vi "ODMR.vi"() -> ()   [LabVIEW 2017]
uses:
  Expose/Labview/Parameters/ExposeParameterBindingType.ctl
  041ffc80-b207-4d08-bfc5-6ab2d64e676f.vi
  451f70a8-fd5b-4474-9a91-34906ede201c.vi
  76a4058a-f0a1-42dc-85a2-e75da8ad429b.vi
  Experiment/ExpGet.vi
  Expose/Labview/Core/ExposeInvokeMethod.vi
  <userlib>/_OpenG.lib/lvdata/lvdata.llb/Get Default Data from Variant__ogtk.vi
panel:
  in  "btnAbort":bool
  in  "btnRunOdmr":bool
  in  "GateDisplay":cluster{"amp":dbl[][], "dt":dbl}
  in  "Results":T1
  in  "ReaderProperties":cluster{"BinsPerFreq":u32, "MaxFreq":dbl}={"BinsPerFreq"=1, "MaxFreq"=100000.0} caption="Reader" {"MaxFreq" min=0.0 step=0.1; "BinsPerFreq" min=1 max=10000}
  in  "ScanProperties":T2={"Start"=2800.0, "End"=2900.0, "N"=6, "Dwell"=10.0, "StepSize"=20.0, "Amplitude"=-30.0, "RepCount"=3} caption="Scan" {"RepCount" min=1 max=10000000; "StepSize" min=0.0 step=0.1; "Dwell" min=0.0 step=0.1; "N" step=1; "End" min=0.0 step=0.1; "Start" min=0.0 step=0.1}
  out "LastBinIndex":dbl format="%_7g"
  out "PendingRepetitionCount":dbl format="%_7g"
  out "BinIndexIndicator":dbl(slide) max=201.0 step=1.0 scale=0.0..1.0
  out "PendingRepIndcator":dbl(slide) max=3.0 step=1.0 scale=0.0..1.0
  out "IsWorking":bool=TRUE
  out "ExpID":string="Exp967f258c607eed45caf40f4c3101458dC" caption="Exp. ID (Debug)"
  out "Results":dbl[](graph) caption="ODMR"
  in  "ReadTickTime":dbl
  out "Stream":dbl[](graph) caption="Counts"
  out "Digital Waveform Graph":digitalwaveform(graph)
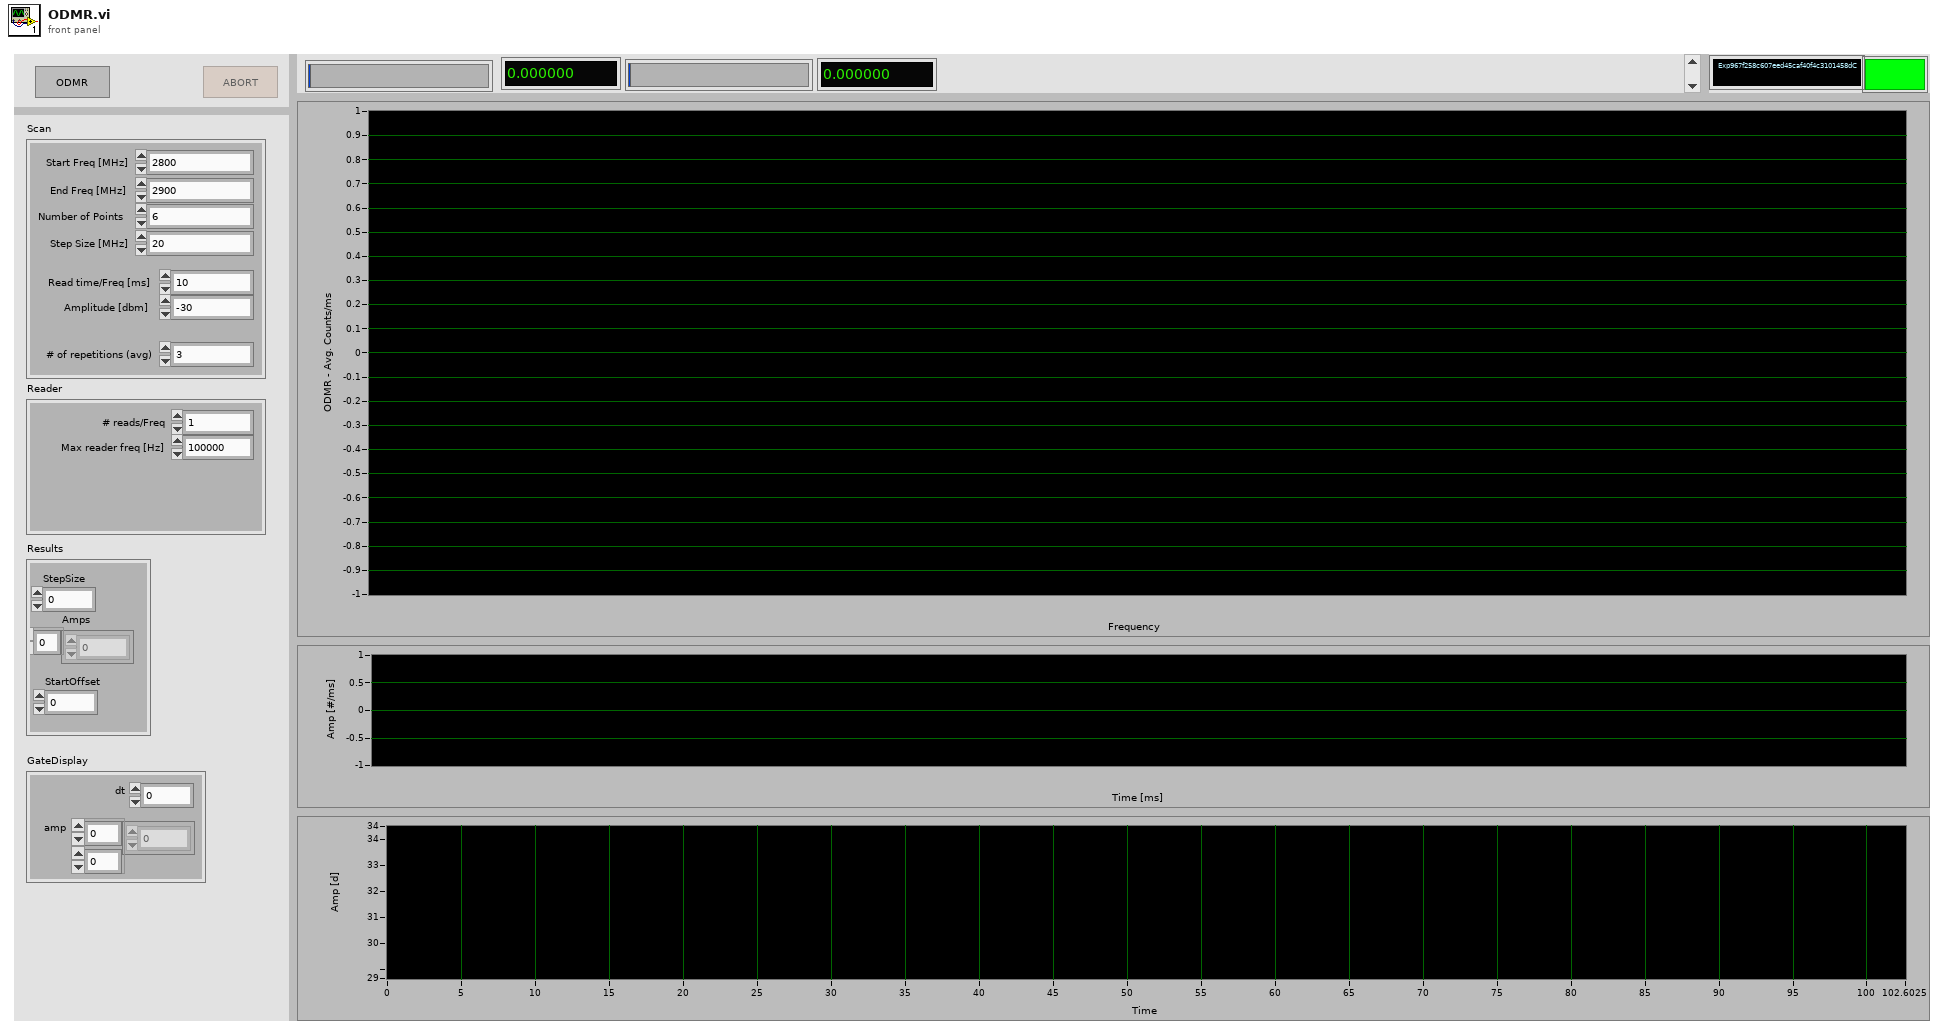
[diagram p1: front panel]
types:
  T1 = cluster{"StepSize":dbl, "Amps":dbl[], "StartOffset":dbl}
  T2 = cluster{"Start":dbl, "End":dbl, "N":u32, "Dwell":dbl, "StepSize":dbl, "Amplitude":dbl, "RepCount":u32}
  T3 = enum8{"Enabled", "Disabled", "Disabled and Grayed Out"}
  T4 = typedef "ExposeParameterBindingType.ctl" = enum16{"ToRemote", "FromRemote", "Bidrectional"}
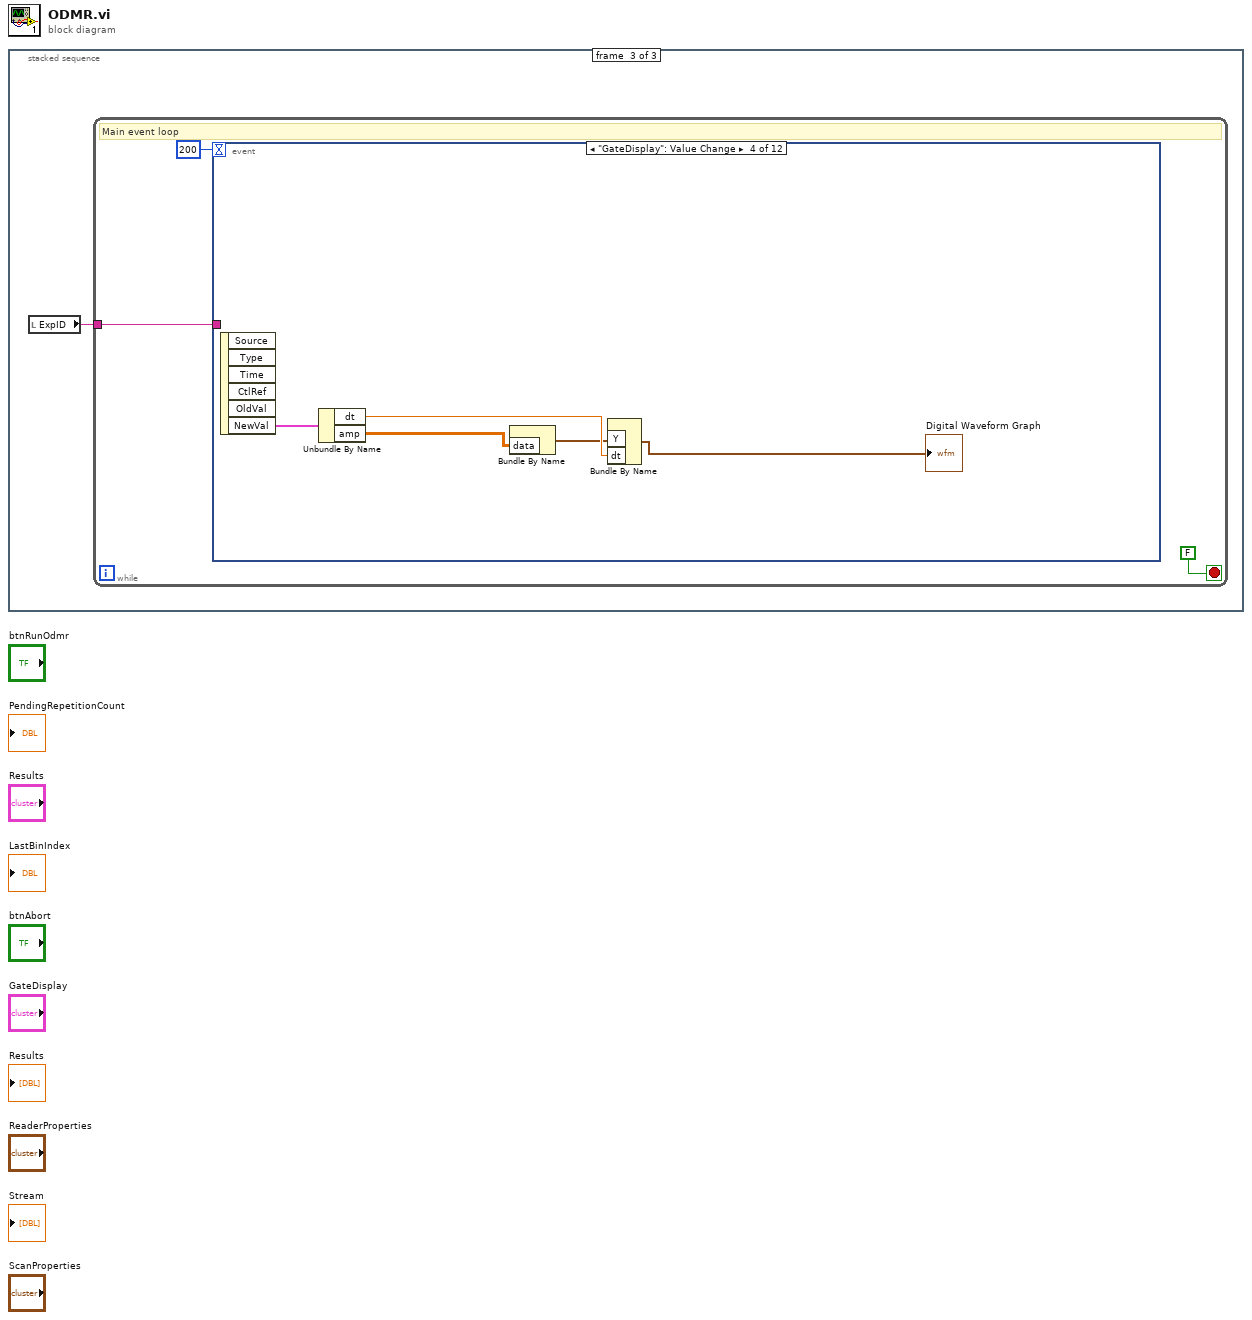
[diagram p0: block diagram]
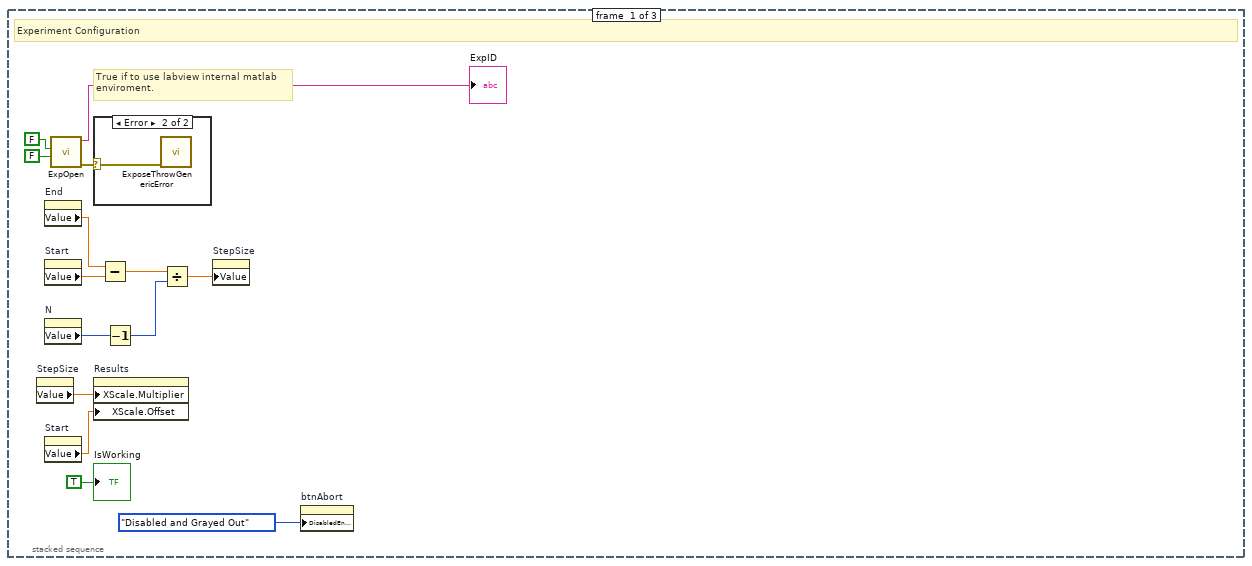
[diagram p2: hidden frame]
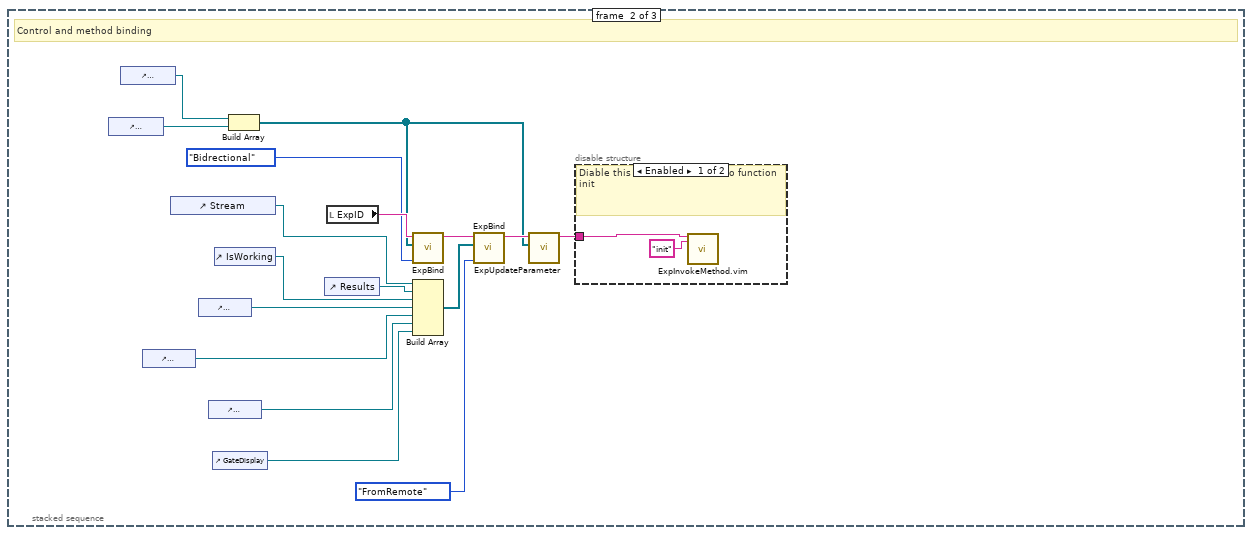
[diagram p4: hidden frame]
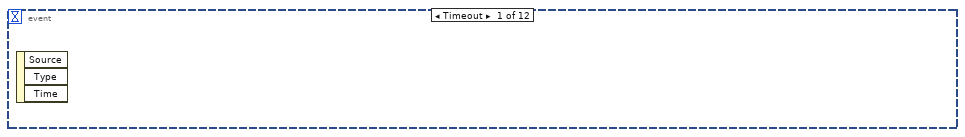
[diagram p6: hidden frame]
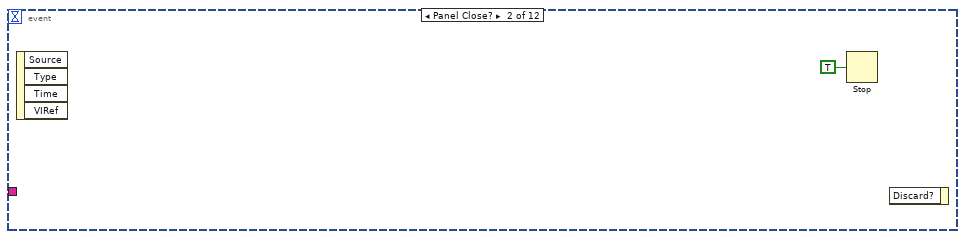
[diagram p7: hidden frame]
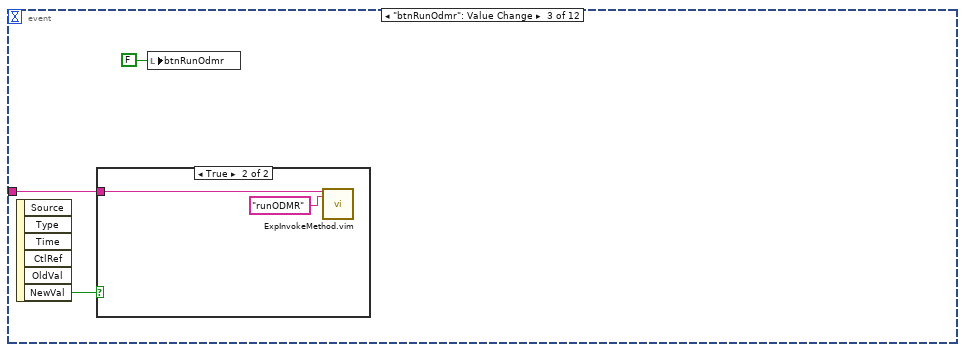
[diagram p8: hidden frame]
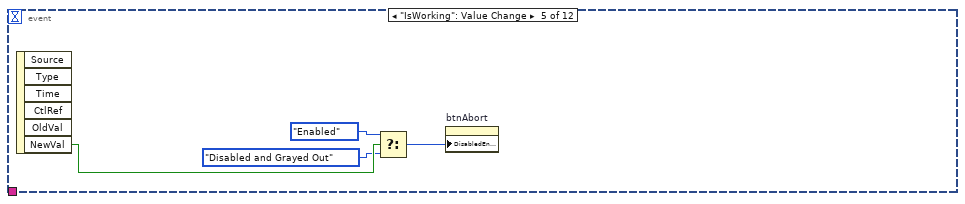
[diagram p10: hidden frame]
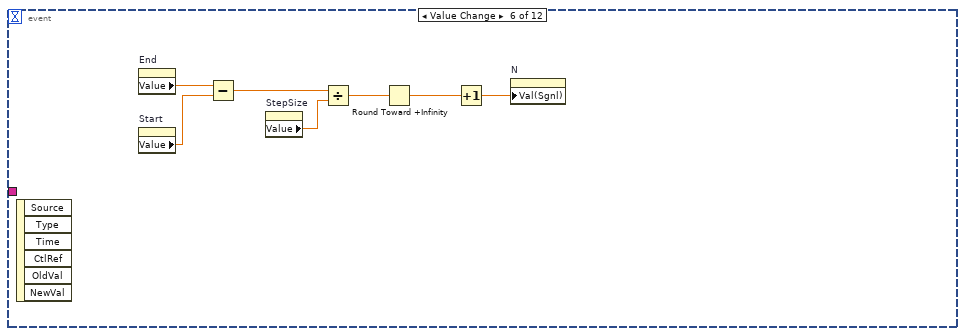
[diagram p11: hidden frame]
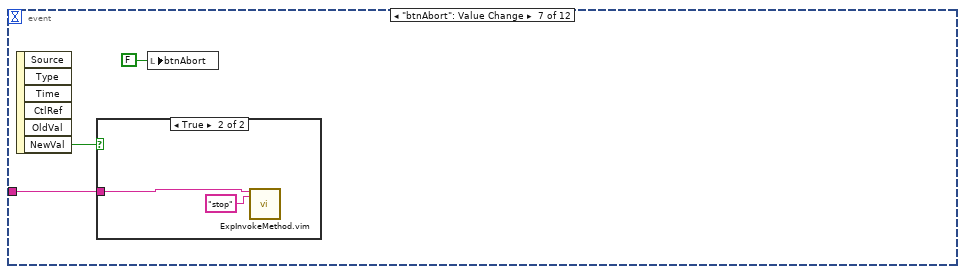
[diagram p12: hidden frame]
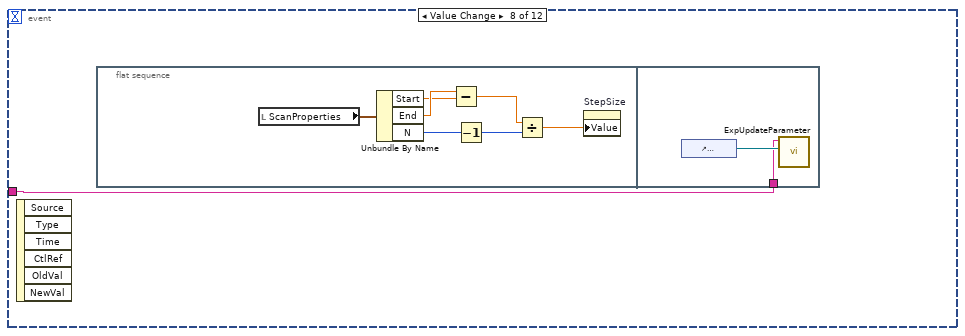
[diagram p14: hidden frame]
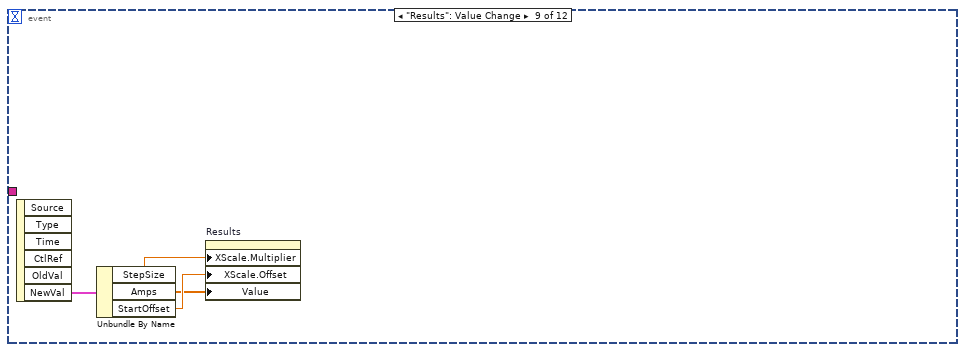
[diagram p15: hidden frame]
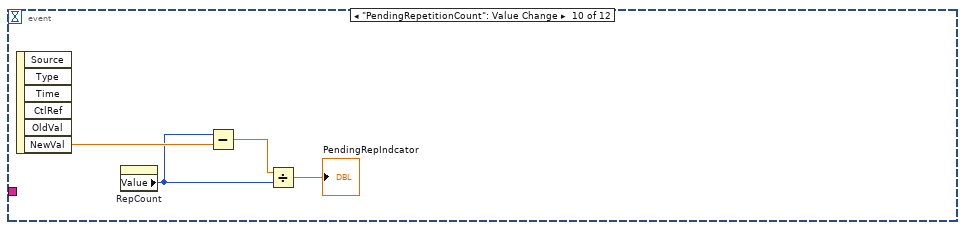
[diagram p16: hidden frame]
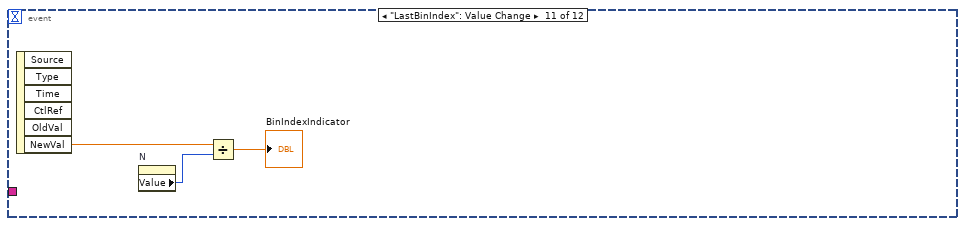
[diagram p17: hidden frame]
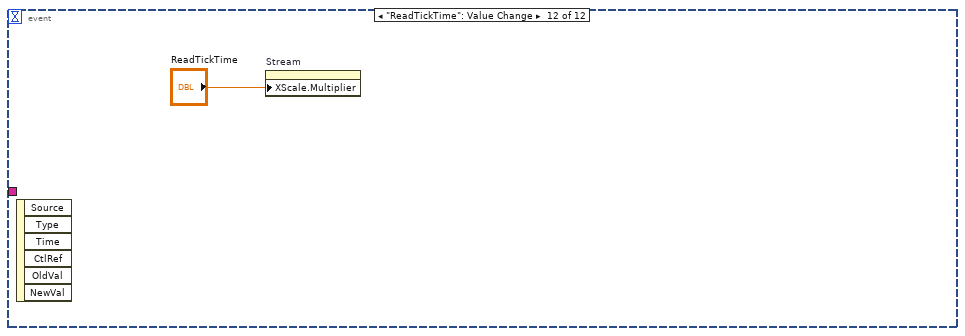
[diagram p18: hidden frame]
diagram:
  n1 = stacked-sequence {
    frame #0 {
      # "True if to use labview internal matlab\nenviroment."
      # "Experiment Configuration"
      n2 = property on="StepSize" class="DigNum (strict)"() -> ("Value"=w2:dbl)  [unwired: 2 in, 2 out]
      n3 = property on="End" class="DigNum (strict)"() -> ("Value"=w10:dbl)  [unwired: 2 in, 2 out]
      n4 = property on="Start" class="DigNum (strict)"() -> ("Value"=w9:dbl)  [unwired: 2 in, 2 out]
      n5 = property on="N" class="DigNum (strict)"() -> ("Value"=w7:u32)  [unwired: 2 in, 2 out]
      n6 = property on="Start" class="DigNum (strict)"() -> ("Value"=w1:dbl)  [unwired: 2 in, 2 out]
      n7 = call "ExpOpen.vi"("Do Expose Logging"=FALSE, "Requires Matlab Enviroment"=FALSE) -> ("error out"=w12:errorcluster, "ExpID"=→"ExpID":string)  [unwired: 7 in, 1 out]
      n8 = case shown="Error" w12 {
        selector: w12 -> [_ w15]
        frame No Error {
        }
        frame Error {
          n9 = call "ExposeThrowGenericError.vi"("error in (no error)"=w15) -> ()  [unwired: 10 in, 1 out]
        }
      }
      n10 = property on="Results" class="WFGraph (strict)"("XScale.Multiplier"=w2, "XScale.Offset"=w1) -> ()  [unwired: 2 in, 2 out]
      n11 = Subtract(x=w10, y=w9) -> (x-y=w8:dbl)
      n12 = Decrement(x=w7) -> (x-1=w5:u32)
      n13 = Divide(x=w8, y=w5) -> (x/y=w6:dbl)
      n14 = property on="StepSize" class="DigNum (strict)"("Value"=w6) -> ()  [unwired: 2 in, 2 out]
      n15 = property on="btnAbort" class="Bool (strict)"("DisabledEnum"=T3."Disabled and Grayed Out" ("Disabled")) -> ()  [unwired: 2 in, 2 out]
      "IsWorking" <- TRUE ("IsWorking")
    }
    frame #1 {
      # "Control and method binding"
      n16 = control-ref of="ReaderProperties"() -> (w23:refnum<vi>)
      n17 = control-ref of="ScanProperties"() -> (w22:refnum<vi>)
      n18 = control-ref of="PendingRepetitionCount"() -> (w18:refnum<vi>)
      n19 = control-ref of="Stream"() -> (w29:refnum<vi>)
      n20 = control-ref of="ReadTickTime"() -> (w21:refnum<vi>)
      n21 = control-ref of="LastBinIndex"() -> (w17:refnum<vi>)
      n22 = control-ref of="GateDisplay"() -> (w16:refnum<vi>)
      n23 = control-ref of="IsWorking"() -> (w27:refnum<vi>)
      n24 = Build Array(w22, w23) -> (w19:refnum<vi>[])
      n25 = control-ref of="Results"() -> (w20:refnum<vi>)
      n26 = local read "ExpID"() -> (w32:string)
      n27 = call "ExpBind.vi"("Binding Type"=ExposeParameterBindingType."Bidrectional", "Value"=w19, "ExpID"=w32) -> ("ExpID out"=w25:string)  [unwired: 7 in, 1 out]
      n28 = Build Array(w29, w20, w27, w21, w18, w17, w16) -> (w28:refnum<vi>[])
      n29 = call "ExpBind.vi"("Binding Type"=ExposeParameterBindingType."FromRemote", "Value"=w28, "ExpID"=w25) -> ("ExpID out"=w24:string)  [unwired: 7 in, 1 out]
      n30 = call "ExpUpdateParameter.vi"("Variant"=w19, "ExpID"=w24) -> ("ExpID out"=w26:string)  [unwired: 8 in, 1 out]
      n31 = disable-structure shown="Enabled" {
        disable-tunnel: w26 -> [w34 _]
        frame Enabled {
          # "Diable this to remove the call to function init"
          n32 = call "ExpInvokeMethod.vim"("ExpID"=w34, "Method Name"="init") -> ()  [unwired: 15 in, 3 out]
        }
        frame Disabled {
        }
      }
    }
    frame #2 {
      n33 = local read "ExpID"() -> (w35:string)
      n34 = while {
        tunnel: w35 -> [w36]
        stop <- FALSE stop-if-true
        # "Main event loop"
        n35 = event shown="[3] \"GateDisplay\": Value Change" {
          selector: _ -> [_ _ _ _ _ _ _ _ _ _ _ _]
          dyn-events: _ -> [_ _ _ _ _ _ _ _ _ _ _ _]
          timeout: 200 -> [_ _ _ _ _ _ _ _ _ _ _ _]
          tunnel: w36 -> [_ _ w42 _ _ _ w62 w66 _ _ _ _]
          event Timeout {
            n36 = event-data() -> ()  [unwired: 1 in, 3 out]
          }
          event Panel Close? {
            n37 = event-data() -> ()  [unwired: 1 in, 4 out]
            n38 = Stop(stop? (T)=TRUE) -> ()
            n39 = event-data() -> ()  [unwired: 2 in, 1 out]
          }
          event "btnRunOdmr": Value Change {
            n40 = event-data() -> ("NewVal"=w41:bool)  [unwired: 1 in, 5 out]
            n41 = case shown="True" w41 {
              tunnel: w42 -> [_ w44]
              frame False {
              }
              frame True {
                n42 = call "ExpInvokeMethod.vim"("ExpID"=w44, "Method Name"="runODMR") -> ()  [unwired: 15 in, 3 out]
              }
            }
            n43 = local write "btnRunOdmr"(FALSE ("btnRunOdmr")) -> ()
          }
          event "GateDisplay": Value Change {
            n44 = event-data() -> ("NewVal"=w49:cluster{"amp":dbl[][], "dt":dbl})  [unwired: 1 in, 5 out]
            n45 = Unbundle By Name(w49) -> ("dt"=w47:dbl, "amp"=w48:dbl[][])
            n46 = Bundle By Name("data"=w48) -> (w46:digitaldata)  [unwired: 1 in]
            n47 = Bundle By Name("Y"=w46, "dt"=w47) -> (→"Digital Waveform Graph":digitalwaveform)  [unwired: 1 in]
          }
          event "IsWorking": Value Change {
            n48 = event-data() -> ("NewVal"=w53:bool)  [unwired: 1 in, 5 out]
            n49 = Select(t=T3."Enabled" ("Disabled"), s=w53, f=T3."Disabled and Grayed Out" ("Disabled")) -> (s? t:f=w50:T3)
            n50 = property on="btnAbort" class="Bool (strict)"("DisabledEnum"=w50) -> ()  [unwired: 2 in, 2 out]
          }
          event "ScanProperties.StepSize": Value Change {
            n51 = event-data() -> ()  [unwired: 1 in, 6 out]
            n52 = property on="End" class="DigNum (strict)"() -> ("Value"=w60:dbl)  [unwired: 2 in, 2 out]
            n53 = property on="Start" class="DigNum (strict)"() -> ("Value"=w59:dbl)  [unwired: 2 in, 2 out]
            n54 = Subtract(x=w60, y=w59) -> (x-y=w58:dbl)
            n55 = property on="StepSize" class="DigNum (strict)"() -> ("Value"=w57:dbl)  [unwired: 2 in, 2 out]
            n56 = Divide(x=w58, y=w57) -> (x/y=w56:dbl)
            n57 = Round Toward +Infinity(x=w56) -> (ceil(x): smallest int >= x=w55:dbl)
            n58 = Increment(x=w55) -> (x+1=w54:dbl)
            n59 = property on="N" class="DigNum (strict)"("Val(Sgnl)"=w54) -> ()  [unwired: 2 in, 2 out]
          }
          event "btnAbort": Value Change {
            n60 = event-data() -> ("NewVal"=w63:bool)  [unwired: 1 in, 5 out]
            n61 = case shown="True" w63 {
              tunnel: w62 -> [_ w65]
              frame False {
              }
              frame True {
                n62 = call "ExpInvokeMethod.vim"("ExpID"=w65, "Method Name"="stop") -> ()  [unwired: 15 in, 3 out]
              }
            }
            n63 = local write "btnAbort"(FALSE ("btnAbort")) -> ()
          }
          event "ScanProperties.N": Value Change {
            n64 = event-data() -> ()  [unwired: 1 in, 6 out]
            n65 = flat-sequence {
              tunnel: w66 -> [w74]
              frame #0 {
                n66 = local read "ScanProperties"() -> (w73:T2)
                n67 = Unbundle By Name(w73) -> ("Start"=w71:dbl, "End"=w72:dbl, "N"=w69:u32)
                n68 = Subtract(x=w72, y=w71) -> (x-y=w70:dbl)
                n69 = Decrement(x=w69) -> (x-1=w67:u32)
                n70 = Divide(x=w70, y=w67) -> (x/y=w68:dbl)
                n71 = property on="StepSize" class="DigNum (strict)"("Value"=w68) -> ()  [unwired: 2 in, 2 out]
              }
              frame #1 {
                n72 = control-ref of="ScanProperties"() -> (w75:refnum<vi>)
                n73 = call "ExpUpdateParameter.vi"("Variant"=w75, "ExpID"=w74) -> ()  [unwired: 8 in, 2 out]
              }
            }
          }
          event "Results": Value Change {
            n74 = event-data() -> ("NewVal"=w79:T1)  [unwired: 1 in, 5 out]
            n75 = Unbundle By Name(w79) -> ("StepSize"=w78:dbl, "Amps"=w76:dbl[], "StartOffset"=w77:dbl)
            n76 = property on="Results" class="WFGraph (strict)"("XScale.Multiplier"=w78, "XScale.Offset"=w77, "Value"=w76) -> ()  [unwired: 2 in, 2 out]
          }
          event "PendingRepetitionCount": Value Change {
            n77 = event-data() -> ("NewVal"=w83:dbl)  [unwired: 1 in, 5 out]
            n78 = property on="RepCount" class="DigNum (strict)"() -> ("Value"=w81:u32)  [unwired: 2 in, 2 out]
            n79 = Subtract(x=w81, y=w83) -> (x-y=w82:dbl)
            n80 = Divide(x=w82, y=w81) -> (x/y=→"PendingRepIndcator":dbl)
          }
          event "LastBinIndex": Value Change {
            n81 = event-data() -> ("NewVal"=w86:dbl)  [unwired: 1 in, 5 out]
            n82 = property on="N" class="DigNum (strict)"() -> ("Value"=w85:u32)  [unwired: 2 in, 2 out]
            n83 = Divide(x=w86, y=w85) -> (x/y=→"BinIndexIndicator":dbl)
          }
          event "ReadTickTime": Value Change {
            n84 = event-data() -> ()  [unwired: 1 in, 6 out]
            n85 = property on="Stream" class="WFGraph (strict)"("XScale.Multiplier"="ReadTickTime") -> ()  [unwired: 2 in, 2 out]
          }
        }
      }
    }
  }
